vi "SRV_Sensor PARSE_##NP.vi"(0 "Return Data":string, 11 "error in (no error)":errorcluster) -> (3 "Sensor View Indicator Names":T1, 10 "Value":dbl, 15 "error out":errorcluster)   [LabVIEW 2009]
uses:
  SRV_Sensors Names.ctl
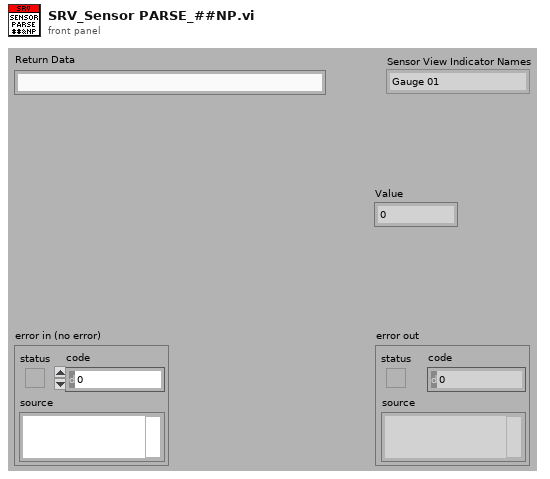
[diagram p1: front panel]
types:
  T1 = typedef "SRV_Sensors Names.ctl" = enum16{"Gauge 01", "Gauge 02", "Gauge 03", "Gauge 04", "Meter 01", "Meter 02", "Meter 03", "Meter 04", "Numeric 01", "Numeric 02", "Numeric 03", "Numeric 04", "Numeric 05", "Numeric 06", "Numeric 07", "Numeric 08", "Boolean 01", "Boolean 02", "Boolean 03", "Boolean 04", "Boolean 05", "Boolean 06", "Boolean 07", "Boolean 08", "Boolean 09", "Boolean 10", "Boolean 11", "Boolean 12", "Boolean 13", "Boolean 14", "Boolean 15", "Boolean 16", "Boolean 17", "Boolean 18", "Boolean 19", "Boolean 20", "Boolean 21", "Boolean 22", "Boolean 23", "Boolean 24", "Boolean 25", "Boolean 26", "Boolean 27", "Boolean 28", "Boolean 29", "Boolean 30", "Boolean 31", "Boolean 32"}
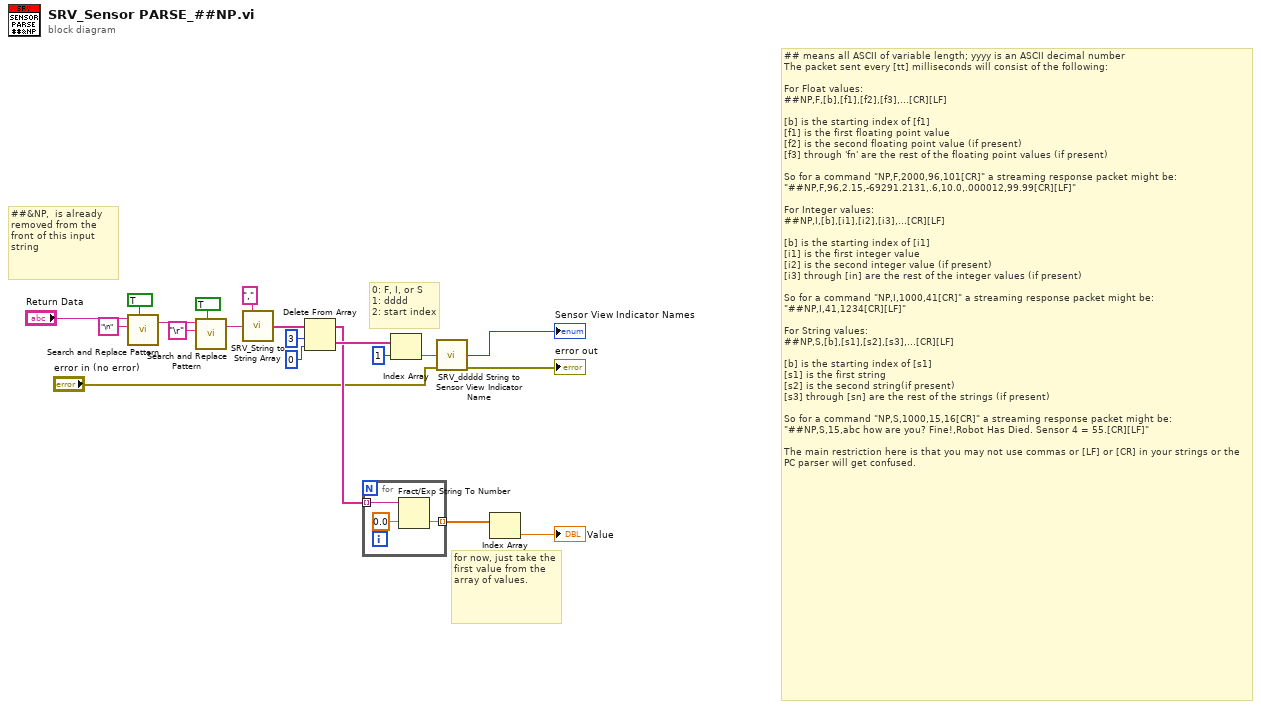
[diagram p0: block diagram]
diagram:
  # "0: F, I, or S\n1: dddd\n2: start index"
  # "for now, just take the first value from the array of values."
  # "##&NP,  is already removed from the front of this input string"
  # "## means all ASCII of variable length; yyyy is an ASCII decimal number\nThe packet sent every [tt] milliseconds will consist of the following:\n\nFor Float values:\n##NP,F,[b],[f1],[f2],[f3],...[CR][LF]\n\n[b] is the starting index of [f1]\n[f1] is the first floating point value\n[f2] is the second floating point value (if present)\n[f3] through 'fn' are the rest of the floating point values (if present)\n\nSo for a command \"NP,F,2000,96,101[CR]\" a streaming response packet might be:\n\"##NP,F,96,2.15,-69291.2131,.6,10.0,.000012,99.99[CR][LF]\"\n\nFor Integer values:\n##NP,I,[b],[i1],[i2],[i3],...[CR][LF]\n\n[b] is the starting index of [i1]\n[i1] is the first integer value\n[i2] is the second integer value (if present)\n[i3] through [in] are the rest of the integer values (if present)\n\nSo for a command \"NP,I,1000,41[CR]\" a streaming response packet might be:\n\"##NP,I,41,1234[CR][LF]\"\n\nFor String values:\n##NP,S,[b],[s1],[s2],[s3],...[CR][LF]\n  \n[b] is the starting index of [s1]\n[s1] is the first string\n[s2] is the second string(if present)\n[s3] through [sn] are the rest of the strings (if present)\n\nSo for a command \"NP,S,1000,15,16[CR]\" a streaming response packet might be:\n\"##NP,S,15,abc how are you? Fine!,Robot Has Died. Sensor 4 = 55.[CR][LF]\"\n\nThe main restriction here is that you may not use commas or [LF] or [CR] in your strings or the PC parser will get confused."
  n1 = call <vilib>:"Search and Replace Pattern.vi"("string"="Return Data", "regular expression (\"\")"="\n" ("regular expression (\"\")"), "replace all? (F)"=TRUE) -> ("result string"=w15:string)  [unwired: 2 in, 1 out]
  n2 = call <vilib>:"Search and Replace Pattern.vi"("string"=w15, "regular expression (\"\")"="\r" ("regular expression (\"\")"), "replace all? (F)"=TRUE) -> ("result string"=w14:string)  [unwired: 2 in, 1 out]
  n3 = call "SRV_String to String Array.vi"("Element Separator (,)"=",", "String"=w14) -> ("String Array"=w12:string[])  [unwired: 13 in]
  n4 = Delete From Array(array=w12, length=3, index=0) -> (deleted portion=w9:string[], array with subset deleted=w8:string[])
  n5 = for {
    tunnel: w8 -> [w23] mode=indexing
    tunnel: [w21] -> w7 mode=indexing
    n6 = Fract/Exp String To Number(string=w23, default (0 dbl)=0.0 ("default (0 DBL)")) -> (number=w21:dbl)  [unwired: 2 in, 1 out]
  }
  n7 = Index Array(array=w9, index=1) -> (element=w3:string)
  n8 = call "SRV_ddddd String to Sensor View Indicator Name.vi"("ddddd"=w3, "error in (no error)"="error in (no error)") -> ("Sensor View Indicator Names"=→"Sensor View Indicator Names":T1, "error out"=→"error out":errorcluster)  [unwired: 12 in]
  n9 = Index Array(array=w7) -> (element=→"Value":dbl)  [unwired: 1 in]
